vi "TestPosition.vi"() -> ()   [LabVIEW 2018]
uses:
  Controls/StageInfo.ctl
panel:
  out "Y":u16
  out "X":u16
  in  "Stage Setup Info":T1
  in  "STEP":bool
  in  "SCAN":bool
  out "Done":bool
  out "X(mm)":dbl
  out "Y(mm)":dbl
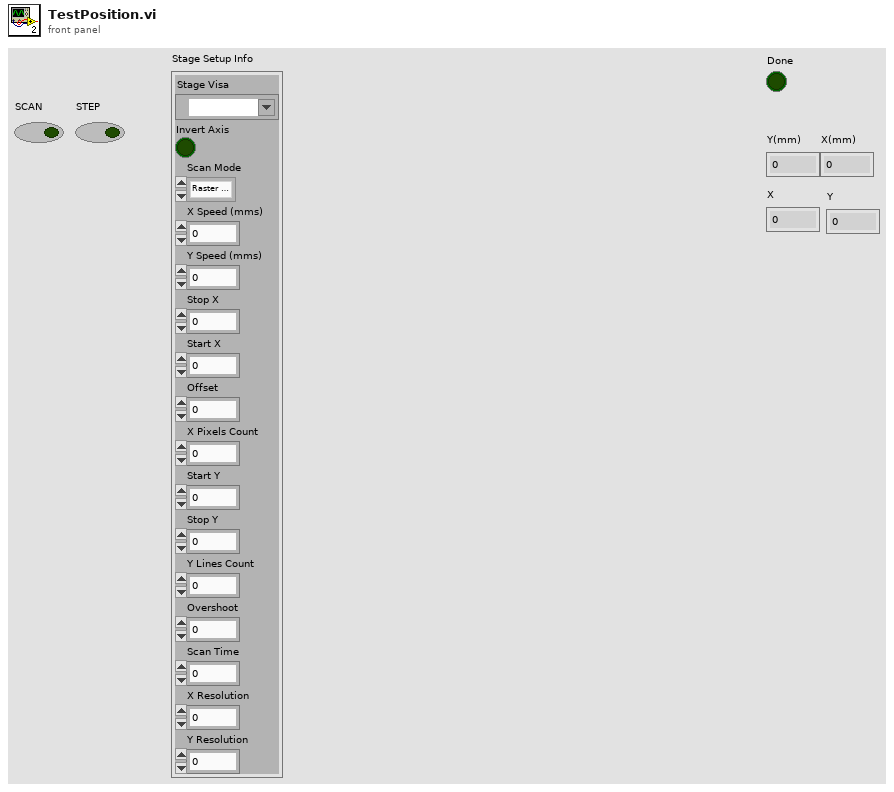
[diagram p1: front panel]
types:
  T1 = typedef "StageInfo.ctl" = cluster{"Stage Visa":refnum<visa-resource-name>, "Invert Axis":bool, "Scan Mode":enum16{"Raster Scan", "Serpentine Scan"}, "X Speed (mms)":dbl, "Y Speed (mms)":dbl, "Stop X":dbl, "Start X":dbl, "Offset":dbl, "X Pixels Count":i32, "Start Y":dbl, "Stop Y":dbl, "Y Lines Count":i32, "Overshoot":dbl, "Scan Time":dbl, "X Resolution":dbl, "Y Resolution":dbl}
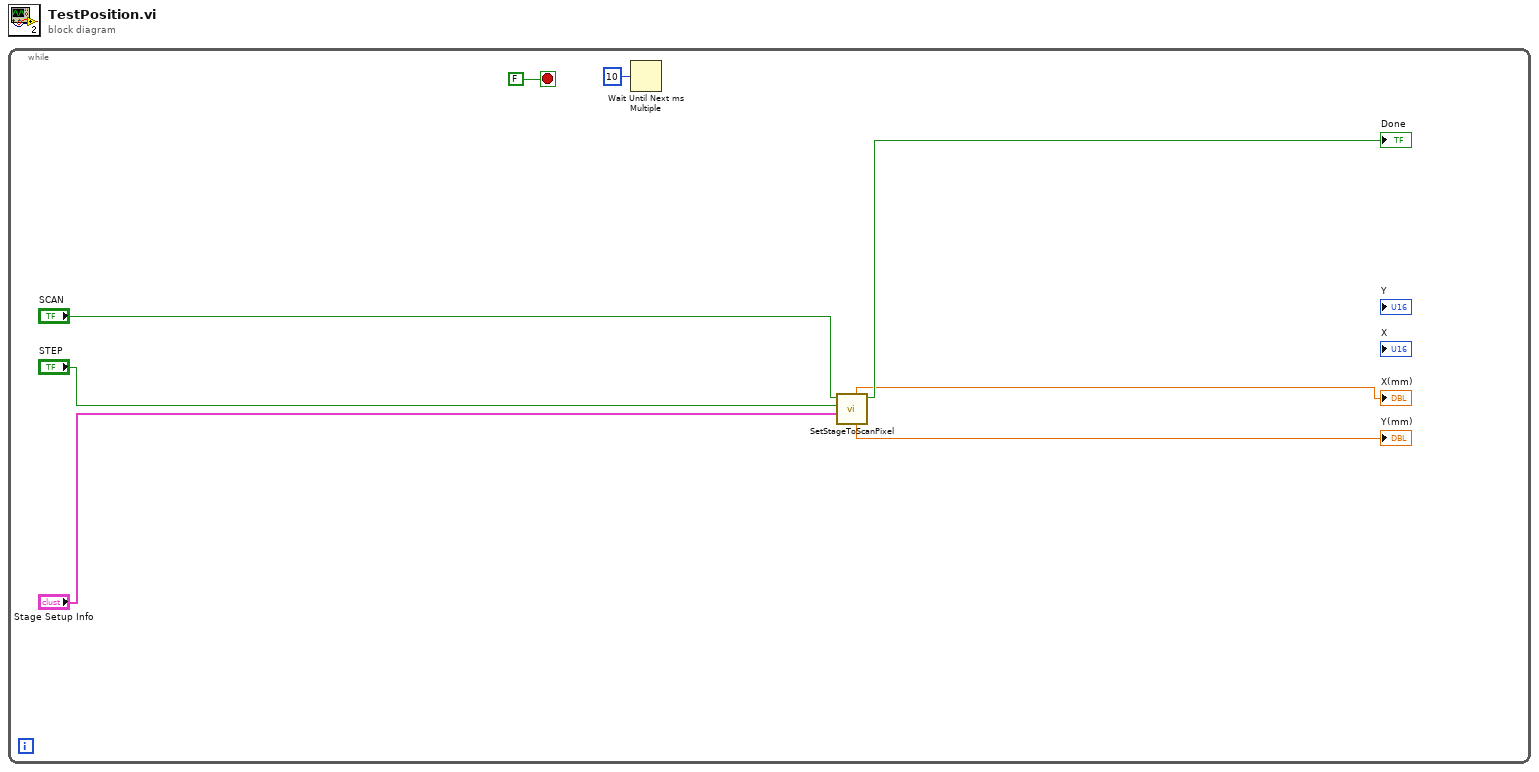
[diagram p0: block diagram]
diagram:
  n1 = while {
    stop <- FALSE stop-if-true
    n2 = Wait Until Next ms Multiple(millisecond multiple=u32 10) -> ()  [unwired: 1 out]
    n3 = call "SetStageToScanPixel.vi"("Stage Setup Info"="Stage Setup Info", "STEP"="STEP", "SCAN"="SCAN") -> ("Completed?"=→"Done":bool, "Y (mm)"=→"Y(mm)":dbl, "X (mm)"=→"X(mm)":dbl)  [unwired: 1 in, 5 out]
  }
